vi "flip flop.vi"(1 "Off":bool, 2 "On":bool, 3 "Pulse":bool) -> (0 "output":bool)   [LabVIEW 2009]
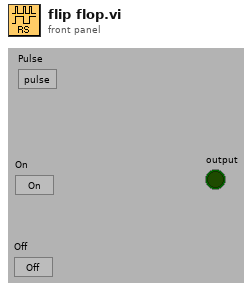
[diagram p1: front panel]
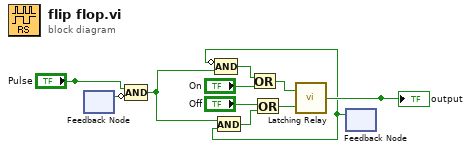
[diagram p0: block diagram]
diagram:
  n1 = feedback #1() -> (w3:bool)  [unwired: 1 in]
  n2 = Compound Arithmetic op=AND("Pulse", invert w3) -> (w1:bool)
  n3 = feedback #2() -> (w4:bool)  [unwired: 1 in]
  n4 = And(x=w1, y=w4) -> (x .and. y?=w6:bool)
  n5 = Compound Arithmetic op=AND(invert w4, w1) -> (w5:bool)
  n6 = Or(x=w5, y="On") -> (x .or. y?=w11:bool)
  n7 = Or(x="Off", y=w6) -> (x .or. y?=w10:bool)
  n8 = call "Latching Relay.vi"("Reset"=w10, "Trigger"=w11) -> ("output"=w7:bool)
  "output" <- w7
